vi "To JSON.vi"(8 "error in":errorcluster, 11 "PDO Slot in":refnum<class "PDO Slot.lvclass">) -> (0 "error out":errorcluster, 2 "JSON":string, 3 "PDO Slot out":refnum<class "PDO Slot.lvclass">)   [LabVIEW 2024, in "PDO Grid.lvlib" / "PDO Slot.lvclass"]
uses:
  PDO Slot.lvclass
  PDO Slot.lvclass/PDO Slot.ctl
  <vilib>/JDP Science/JSONtext/Get all Object Items.vi
  <vilib>/JDP Science/JSONtext/Set Multiple Object Items.vi
  Core/PDO Communication Parameter/PDO Communication Parameter.lvclass
  PDO Mapping/PDO Mapping.lvclass
  <vilib>/JDP Science/JSONtext/JSONtext.lvlib
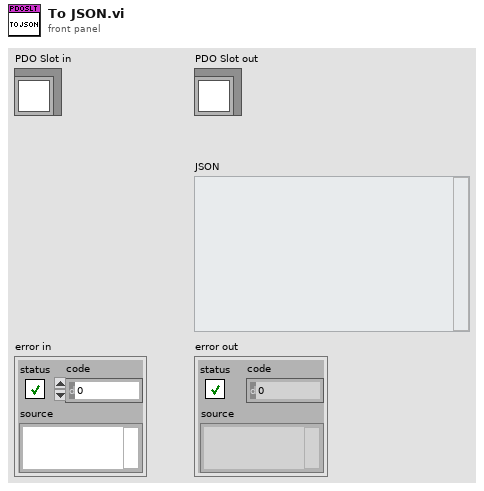
[diagram p1: front panel]
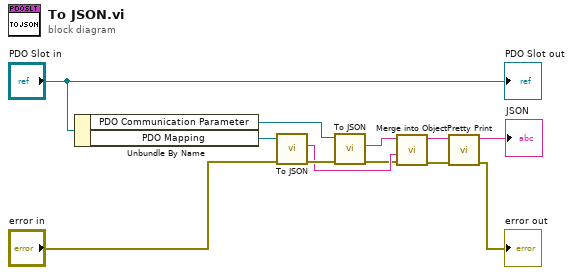
[diagram p0: block diagram]
diagram:
  n1 = Unbundle By Name("PDO Slot in") -> ("PDO Communication Parameter"=w11:refnum<class "PDO Communication Parameter.lvclass">, "PDO Mapping"=w8:refnum<class "PDO Mapping.lvclass">)
  n2 = call "To JSON.vi"("error in"="error in", "PDO Mapping in"=w8) -> ("error out"=w9:errorcluster, "<JSON>"=w7:string)  [unwired: 7 in, 1 out]
  n3 = call "To JSON.vi"("error in"=w9, "PDO Communication Parameter in"=w11) -> ("error out"=w5:errorcluster, "<JSON>"=w6:string)  [unwired: 7 in, 1 out]
  n4 = call <vilib>:"Merge into Object.vi"("error in (no error)"=w5, "JSON Object to Merge"=w7, "JSON"=w6) -> ("error out"=w4:errorcluster, "<JSON>"=w2:string)  [unwired: 6 in]
  n5 = call <vilib>:"Pretty Print.vi"("error in (no error)"=w4, "JSON"=w2) -> ("error out"=→"error out":errorcluster, "<JSON>"=→"JSON":string)  [unwired: 7 in, 1 out]
  "PDO Slot out" <- "PDO Slot in"
